vi "Output Enable Write Single.vi"(8 "error in":errorcluster, 9 "Channel Index":i32=1, 10 "Output Enable STS":i32, 11 "Cycler in":refnum<class "Cycler.lvclass">) -> (0 "error out":errorcluster, 3 "Cycler out":refnum<class "Cycler.lvclass">)   [LabVIEW 2023, in "Cycler.lvclass"]
uses:
  Cycler.lvclass
  Cycler.lvclass/Cycler.ctl
  Low Level Capabilities/Output Enable/Output Enable.lvclass
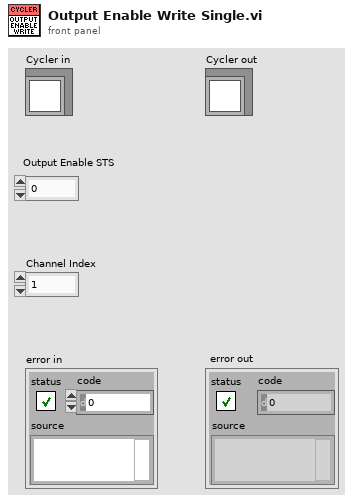
[diagram p1: front panel]
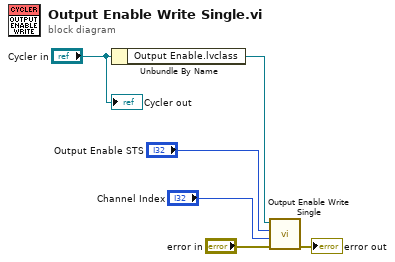
[diagram p0: block diagram]
diagram:
  n1 = Unbundle By Name("Cycler in") -> ("Output Enable.lvclass"=w2:refnum<class "Output Enable.lvclass">)
  n2 = call-dynamic "Output Enable Write Single.vi"("error in"="error in", "Channel Index"="Channel Index", "Output Enable STS"="Output Enable STS", "Output Enable in"=w2) -> ("error out"=→"error out":errorcluster)  [unwired: 6 in, 1 out]
  "Cycler out" <- "Cycler in"
